vi "Get Strings from Ref.vi"(8 "error in (no error)":errorcluster, 9 "Label Prefix":string, 10 "GObj Refnum in":refnum<vi>, 11 "GObject in":refnum<class "GObject.lvclass">) -> (0 "error out":errorcluster, 1 "Valid?":bool, 2 "GObj Refnum out":refnum<vi>, 3 "GObject out":refnum<class "GObject.lvclass">, 4 "GObj Name":string)   [LabVIEW 2013, in "SET Project Data.lvlib" / "GObject.lvclass"]
uses:
  GObject.lvclass
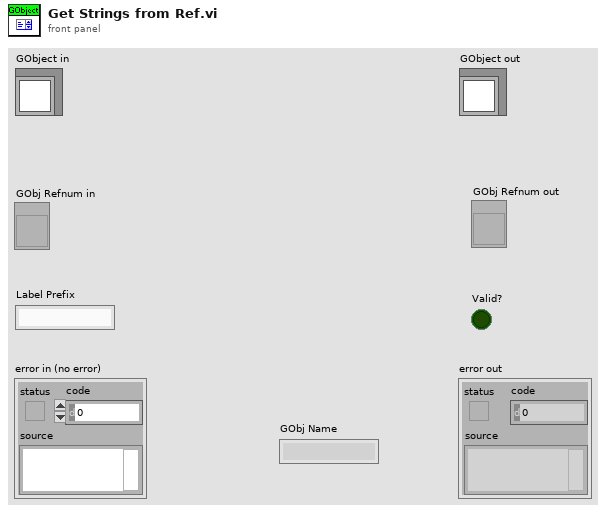
[diagram p1: front panel]
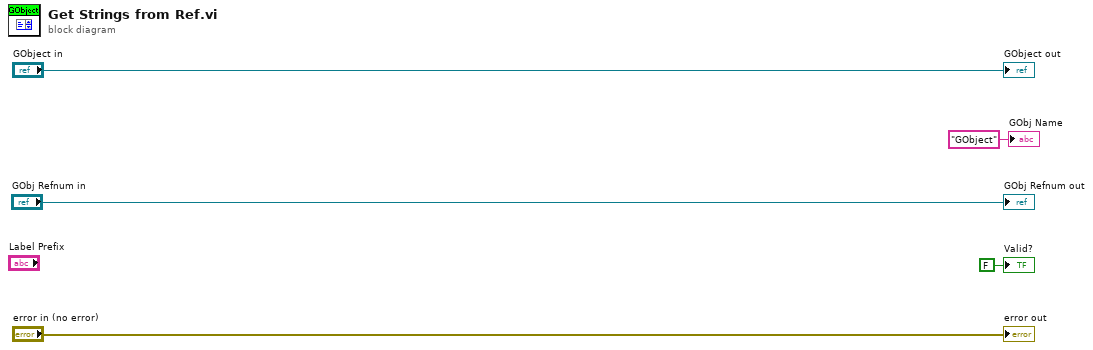
[diagram p0: block diagram]
diagram:
  "error out" <- "error in (no error)"
  "GObject out" <- "GObject in"
  "GObj Refnum out" <- "GObj Refnum in"
  "Valid?" <- FALSE ("Valid?")
  "GObj Name" <- "GObject" ("Control Name")
